vi "Get Required Driver Types.vi"(8 "error in (no error)":errorcluster, 11 "Custom Multi Instrument Msg in":refnum<class "Custom Multi Instrument Msg.lvclass">) -> (0 "error out":errorcluster, 2 "Required Driver Types":T1[](array[typedef]), 3 "Custom Multi Instrument Msg out":refnum<class "Custom Multi Instrument Msg.lvclass">)   [LabVIEW 2020, in "Instrument Handler.lvlib" / "Custom Multi Instrument Msg.lvclass"]
doc: "Get the Required Driver Types and count of each driver for execution of the Instrument Msg."
uses:
  Custom Multi Instrument Msg.lvclass
  Messages/Multi Instrument Msg/Ctl_RequiredInstrumentElement.ctl
  PPL/HDH.Actor Framework.Core.Instrument Driver.lvlibp/Instrument Driver/Instrument Driver.lvclass
  Messages/Instrument Msg/Instrument Msg.lvclass
  Messages/Multi Instrument Msg/Multi Instrument Msg.lvclass
  Custom Multi Instrument Msg.lvclass/Custom Multi Instrument Msg.ctl
  PPL/HDH.Actor Framework.Core.Actor.lvlibp/1abvi3w/vi.lib/ActorFramework/Message/Message.lvclass
  PPL/HDH.Actor Framework.Core.Sequencer.lvlibp
  PPL/HDH.Data.Generic.lvlibp
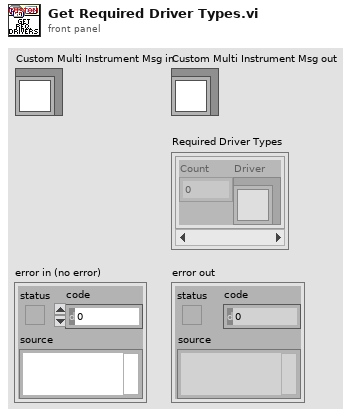
[diagram p1: front panel]
types:
  T1 = typedef "Instrument Handler.lvlib/Multi Instrument Msg.lvclass/Ctl_RequiredInstrumentElement.ctl" = cluster{"Count":i16, "Driver":refnum<class "Instrument Driver.lvclass">}
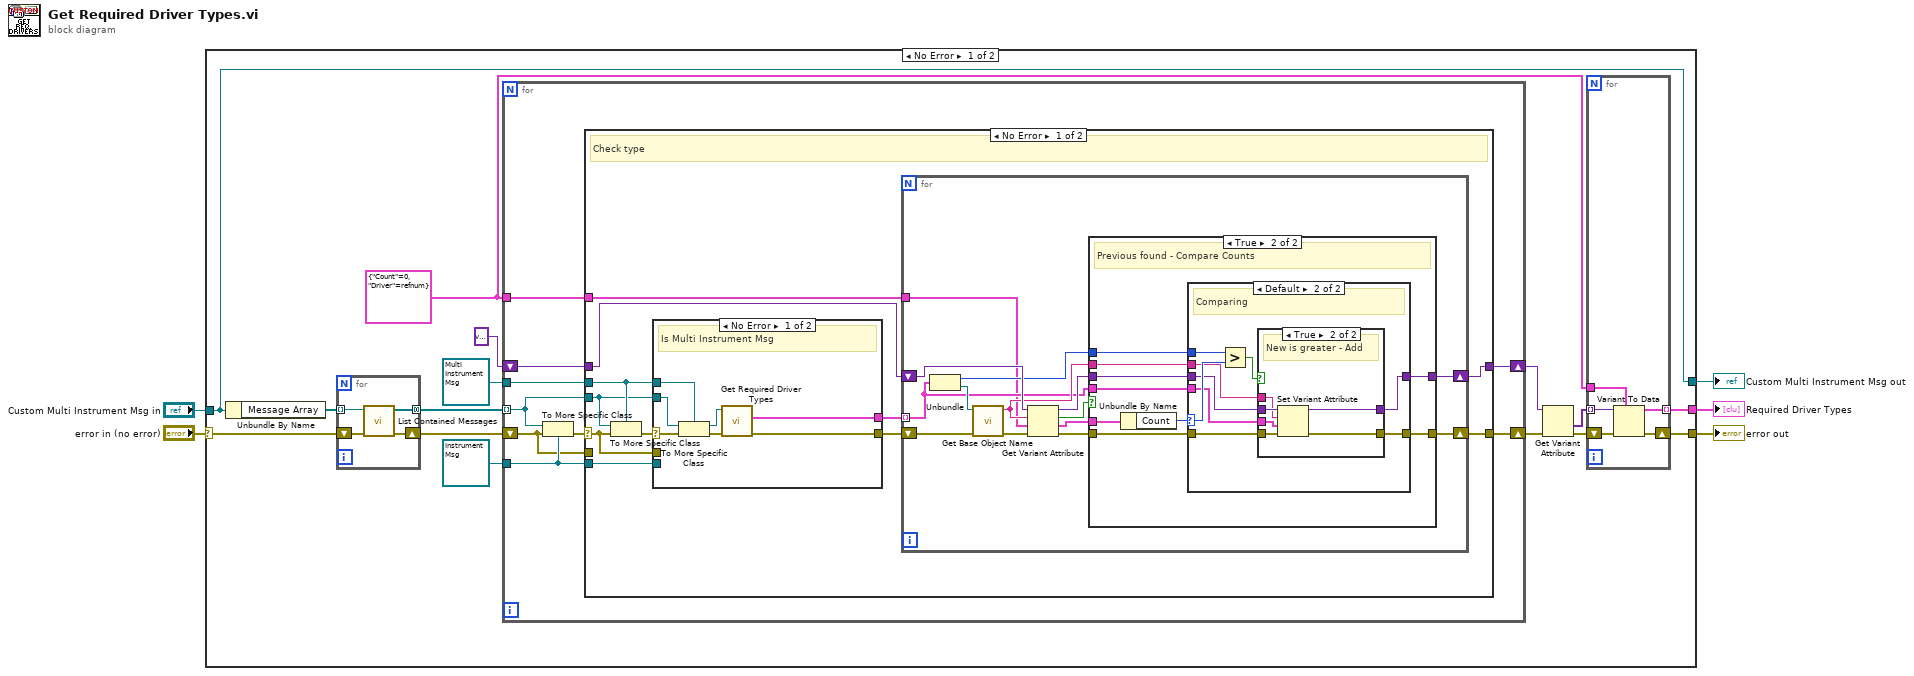
[diagram p0: block diagram]
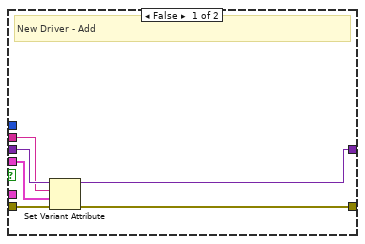
[diagram p2: hidden frame]
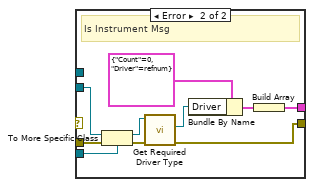
[diagram p5: hidden frame]
diagram:
  n1 = case shown="No Error" "error in (no error)" {
    selector: "error in (no error)" -> [w7 w118]
    tunnel: "Custom Multi Instrument Msg in" -> [w17 w117]
    tunnel: [w10 w118] -> w3
    tunnel: [w17 w117] -> w2
    tunnel: [w12 _] -> w1
    frame No Error {
      w13 = T1 {"Count"=0, "Driver"=refnum} ("Required Driver Types")
      n2 = Unbundle By Name(w17) -> ("Message Array"=w9:refnum<class "Message.lvclass">[])
      n3 = for {
        tunnel: w9 -> [w24] mode=indexing
        shift-right: [w22] -> w6
        shift-left: w7 -> [w23]
        tunnel: [w21] -> w8 mode=concatenating
        n4 = call "List Contained Messages.vi"("error in (no error)"=w23, "Message"=w24) -> ("error out"=w22:errorcluster, "Message Array"=w21:refnum<class "Message.lvclass">[])  [unwired: 8 in]
      }
      n5 = for {
        tunnel: w8 -> [w35] mode=indexing
        tunnel: refnum<class "Instrument Msg.lvclass"> refnum ("Instrument Handler.lvlib:Instrument Msg.lvclass") -> [w33]
        shift-right: [w37] -> w16
        shift-left: variant -> [w36]
        tunnel: refnum<class "Multi Instrument Msg.lvclass"> refnum ("Instrument Handler.lvlib:Multi Instrument Msg.lvclass") -> [w34]
        shift-right: [w32] -> w15
        shift-left: w6 -> [w30]
        tunnel: w13 -> [w31]
        n6 = To More Specific Class(target class=w33, reference=w35, error in=w30) -> (error out=w38:errorcluster)  [unwired: 1 out]
        n7 = case shown="No Error" w38 {
          selector: w38 -> [w48 _]
          tunnel: [w41 w116] -> w37
          tunnel: w36 -> [w44 w116]
          tunnel: w35 -> [w46 _]
          tunnel: w34 -> [w47 _]
          tunnel: w33 -> [w45 _]
          tunnel: [w40 w115] -> w32
          tunnel: w31 -> [w39 _]
          tunnel: w30 -> [_ w115]
          frame No Error {
            # "Check type"
            n8 = To More Specific Class(target class=w47, reference=w46, error in=w48) -> (error out=w49:errorcluster)  [unwired: 1 out]
            n9 = case shown="No Error" w49 {
              selector: w49 -> [w104 _]
              tunnel: w48 -> [_ w114]
              tunnel: w47 -> [w103 _]
              tunnel: w46 -> [w102 w113]
              tunnel: w45 -> [_ w112]
              tunnel: [w99 w106] -> w43
              tunnel: [w98 w105] -> w42
              frame No Error {
                # "Is Multi Instrument Msg"
                n10 = To More Specific Class(target class=w103, reference=w102, error in=w104) -> (specific class reference=w101:refnum<class "Multi Instrument Msg.lvclass">, error out=w100:errorcluster)
                n11 = call-dynamic "Get Required Driver Types.vi"("error in (no error)"=w100, "Multi Instrument Msg in"=w101) -> ("error out"=w98:errorcluster, "Required Driver Types"=w99:T1[])  [unwired: 7 in, 1 out]
              }
              frame Error {
                # "Is Instrument Msg"
                n12 = To More Specific Class(target class=w112, reference=w113, error in=w114) -> (specific class reference=w111:refnum<class "Instrument Msg.lvclass">, error out=w110:errorcluster)
                n13 = call-dynamic "Get Required Driver Type.vi"("error in (no error)"=w110, "Instrument Msg in"=w111) -> ("error out"=w105:errorcluster, "Required Driver Type"=w108:refnum<class "Instrument Driver.lvclass">)  [unwired: 7 in, 1 out]
                n14 = Bundle By Name(cluster=T1 {"Count"=0, "Driver"=refnum} ("Required Driver Types"), "Driver"=w108) -> (w107:T1)
                n15 = Build Array(w107) -> (w106:T1[])
              }
            }
            n16 = for {
              shift-right: [w61] -> w41
              shift-left: w44 -> [w63]
              tunnel: w43 -> [w57] mode=indexing
              shift-right: [w53] -> w40
              shift-left: w42 -> [w56]
              tunnel: w39 -> [w50]
              n17 = Unbundle(w57) -> ("Count"=w51:i16, "Driver"=w62:refnum<class "Instrument Driver.lvclass">)
              n18 = call "Get Base Object Name.vi"("error in (no error)"=w56, "Object in"=w62) -> ("error out"=w55:errorcluster, "Base class name"=w58:string)  [unwired: 8 in]
              n19 = Get Variant Attribute(Variant=w63, name=w58, default value (empty Variant)=w50, error in=w55) -> (duplicate Variant=w60:variant, found=w59:bool, value=w52:T1, error out=w54:errorcluster)
              n20 = case shown="True" w59 {
                tunnel: [w66 w75] -> w61
                tunnel: w60 -> [w69 w74]
                tunnel: w58 -> [w68 w71]
                tunnel: w57 -> [w67 w70]
                tunnel: w54 -> [w65 w72]
                tunnel: [w64 w73] -> w53
                tunnel: w52 -> [_ w77]
                tunnel: w51 -> [_ w76]
                frame False {
                  # "New Driver - Add"
                  n21 = Set Variant Attribute(Variant=w69, name=w68, value=w67, error in=w65) -> (Variant out=w66:variant, error out=w64:errorcluster)  [unwired: 1 out]
                }
                frame True {
                  # "Previous found - Compare Counts"
                  n22 = Unbundle By Name(w77) -> ("Count"=w78:i16)
                  n23 = case shown="Default" w78 {
                    selector: w78 -> [_ w88]
                    tunnel: w76 -> [_ w89]
                    tunnel: [w80 w86] -> w75
                    tunnel: w74 -> [w80 w85]
                    tunnel: [w79 w84] -> w73
                    tunnel: w72 -> [w79 w83]
                    tunnel: w71 -> [_ w82]
                    tunnel: w70 -> [_ w81]
                    frame -1 {
                      # "Largest count already set"
                    }
                    frame Default {
                      # "Comparing"
                      n24 = Greater?(x=w89, y=w88) -> (0:w87:bool)
                      n25 = case shown="True" w87 {
                        tunnel: [w91 w96] -> w86
                        tunnel: w85 -> [w91 w97]
                        tunnel: [w90 w94] -> w84
                        tunnel: w83 -> [w90 w95]
                        tunnel: w82 -> [_ w93]
                        tunnel: w81 -> [_ w92]
                        frame False {
                          # "Don't add"
                        }
                        frame True {
                          # "New is greater - Add"
                          n26 = Set Variant Attribute(Variant=w97, name=w93, value=w92, error in=w95) -> (Variant out=w96:variant, error out=w94:errorcluster)  [unwired: 1 out]
                        }
                      }
                    }
                  }
                }
              }
            }
          }
          frame Error {
            # "No required Instruments"
          }
        }
      }
      n27 = Get Variant Attribute(Variant=w16, error in=w15) -> (values=w14:variant[], error out=w11:errorcluster)  [unwired: 2 in, 2 out]
      n28 = for {
        tunnel: w14 -> [w29] mode=indexing
        tunnel: w13 -> [w28]
        tunnel: [w27] -> w12 mode=indexing
        shift-right: [w25] -> w10
        shift-left: w11 -> [w26]
        n29 = Variant To Data(error in=w26, type=w28, Variant=w29) -> (data=w27:T1, error out=w25:errorcluster)
      }
    }
    frame Error {
    }
  }
  "error out" <- w3
  "Custom Multi Instrument Msg out" <- w2
  "Required Driver Types" <- w1
